vi "Meter Randomize Infos.vi"(10 "DeviceID":T2) -> (3 "Meter_Info Array out":T1[](array[typedef]))   [LabVIEW 2018, in "IED Test Framework.lvlib" / "IED Test.lvclass"]
uses:
  IED Test.lvclass
  <vilib>/ORNL/CSEISMIC DDS/CSEISMIC DDS Base/Data Types/Controls/DeviceID.ctl
  <vilib>/ORNL/CSEISMIC DDS/CSEISMIC DDS Base/Data Types/Meter_Info.ctl
  <vilib>/ORNL/CSEISMIC DDS/CSEISMIC DDS Base/CSEISMIC DDS.lvclass
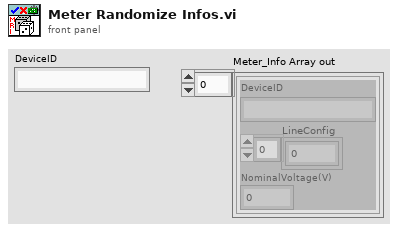
[diagram p1: front panel]
types:
  T1 = typedef "CSEISMIC DDS.lvlib/CSEISMIC DDS.lvclass/Meter_Info.ctl" = cluster{"DeviceID":T2, "LineConfig":u8[], "NominalVoltage(V)":dbl}
  T2 = typedef "CSEISMIC DDS.lvlib/CSEISMIC DDS.lvclass/DeviceID.ctl" = string
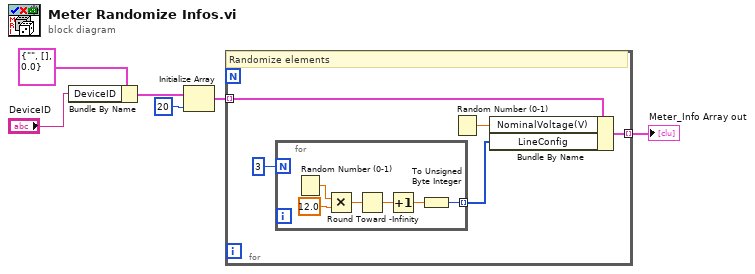
[diagram p0: block diagram]
diagram:
  n1 = Bundle By Name(cluster=T1 {"DeviceID"="", "LineConfig"=[], "NominalVoltage(V)"=0.0} ("Meter_Measurement Array out"), "DeviceID"="DeviceID") -> (w6:T1)
  n2 = Initialize Array(w6, 20 ("dimension size")) -> (w3:T1[])
  n3 = for {
    tunnel: w3 -> [w11] mode=indexing
    tunnel: [w10] -> w1 mode=indexing
    # "Randomize elements"
    n4 = for {
      N: 3 -> [_]
      tunnel: [w13] -> w8 mode=indexing
      n5 = Random Number (0-1)() -> (number: 0 to 1=w17:dbl)
      n6 = Multiply(x=w17, y=12.0) -> (x*y=w15:dbl)
      n7 = Round Toward -Infinity(1:w15) -> (0:w14:dbl)
      n8 = Increment(x=w14) -> (x+1=w12:dbl)
      n9 = To Unsigned Byte Integer(number=w12) -> (unsigned 8bit integer=w13:u8)
    }
    n10 = Random Number (0-1)() -> (number: 0 to 1=w7:dbl)
    n11 = Bundle By Name(cluster=w11, "NominalVoltage(V)"=w7, "LineConfig"=w8) -> (w10:T1)
  }
  "Meter_Info Array out" <- w1
